vi "Send_User_Event.vi"(6 "priority (normal)":T1=enum."normal priority", 8 "error in (no error)":errorcluster, 9 "Data":variant, 10 "Command":string, 11 "user event In":refnum<user-event>) -> (0 "error out":errorcluster, 3 "user event Out":refnum<user-event>)   [LabVIEW 2014, in "User_Event_Library.lvlib"]
uses:
  User_Event_Library.lvlib
  TypeDef.ctl
  <vilib>/event_ctls.llb/usereventprio.ctl
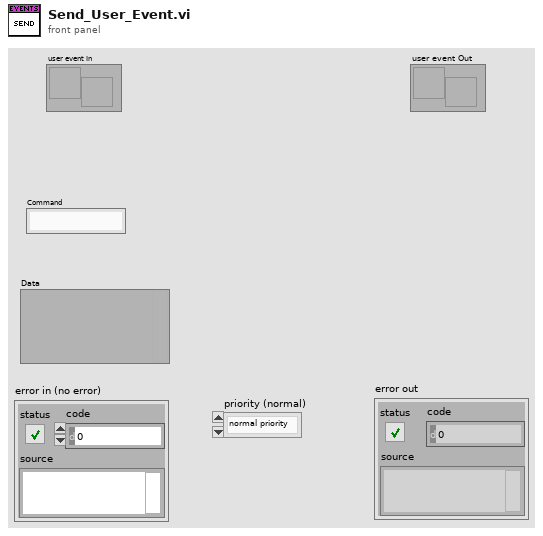
[diagram p1: front panel]
types:
  T1 = typedef "usereventprio.ctl" = enum32{"high priority", "normal priority"}
  T2 = typedef "User_Event_Library.lvlib/TypeDef.ctl" = cluster{"Command":string, "Data":variant}
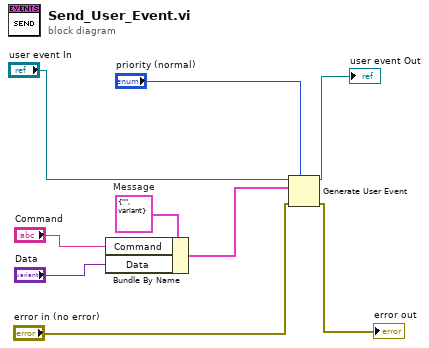
[diagram p0: block diagram]
diagram:
  w9 = T2 {"Command"="", "Data"=variant}  # Message
  n1 = Bundle By Name(cluster=w9, "Command"="Command", "Data"="Data") -> (w5:T2)
  n2 = Generate User Event(priority (normal)="priority (normal)", user event="user event In", event data cluster=w5, error in="error in (no error)") -> (user event out=→"user event Out":refnum<user-event>, error out=→"error out":errorcluster)
